vi "LH-01-17.vi"(0 "FPGA VI Reference In":refnum<k20>, 1 "OutputRange":cluster{"output high":dbl, "output low":dbl}[](array[cluster]), 2 "LHSetpoints":dbl[](array[numeric]), 3 "AIsLH":i32[](array[numeric]), 4 "error in":errorcluster, 6 "PIDs für \"träge\" Heizungen":T1(array[cluster])) -> (7 "error out":errorcluster)   [LabVIEW 2010]
uses:
  <vilib>/rvi/interface/nirviReadWriteControl/nirviReadWriteControl.xnode
  C:/Users/HAGAR-IV/Desktop/Zeugs/markus/version feb 2012/FPGA Bitfiles/pertrasgcfpga2_FPGATarget_FPGA-Programm-01_A75D3647.lvbitx
  C:/Users/HAGAR-IV/Desktop/Zeugs/Johnny/pertrasgc fpga/FPGA-Programm-01-17.vi
  <vilib>/rvi/interface/common/niFpgaNodeNameForErrorReporting.ctl
  <vilib>/rvi/errors/niLvFpgaWhatHappensToTopLevelVI.ctl
  GVHeizenLH.vi
  GVAIs.vi
  <vilib>/addons/control/pid/pid.llb/PID (DBL Array).vi
  <vilib>/Utility/error.llb/Error Cluster From Error Code.vi
  <vilib>/rvi/errors/niLvFpgaAdjustHostInterfaceError.vi
  <vilib>/addons/control/pid/NI_PID_pid.lvlib
  NiFpgaLv.dll
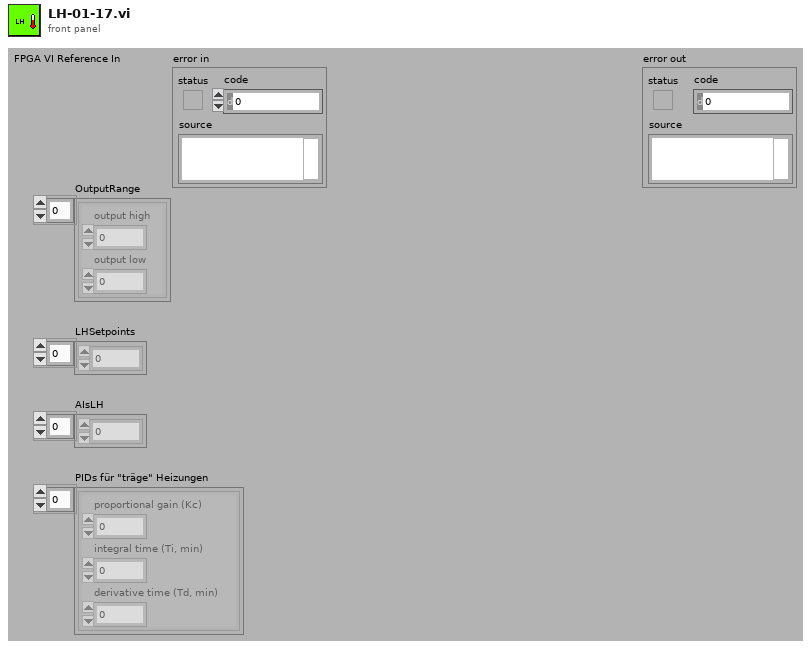
[diagram p1: front panel]
types:
  T1 = cluster{"proportional gain (Kc)":dbl, "integral time (Ti, min)":dbl, "derivative time (Td, min)":dbl}[]
  T2 = cluster{"Heizen?LH[0]":bool, "Heizen?LH[1]":bool, "Heizen?LH[2]":bool, "Heizen?LH[3]":bool, "Heizen?LH[4]":bool, "Heizen?LH[5]":bool, "Heizen?LH[6]":bool, "Heizen?LH[7]":bool, "Heizen?LH[8]":bool, "Heizen?LH[9]":bool, "Heizen?LH[10]":bool, "Heizen?LH[11]":bool}
  T3 = cluster{"[0]":u32, "[1]":u32, "[2]":u32, "[3]":u32, "[4]":u32, "[5]":u32, "[6]":u32, "[7]":u32, "[8]":u32, "[9]":u32, "[10]":u32, "[11]":u32}
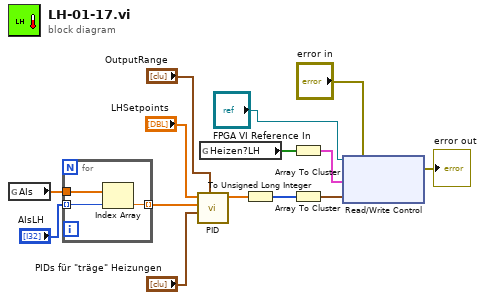
[diagram p0: block diagram]
diagram:
  n1 = global read "GVAIs.vi" "AIs"() -> (w12:dbl[])
  n2 = for {
    tunnel: w12 -> [w17]
    tunnel: "AIsLH" -> [w16] mode=indexing
    tunnel: [w15] -> w1 mode=indexing
    n3 = Index Array(array=w17, index=w16) -> (element=w15:dbl)
  }
  n4 = call-poly <vilib>:"PID.vi"("output range"="OutputRange", "PID gains"="PIDs für \"träge\" Heizungen", "process variable"=w1, "setpoint"="LHSetpoints") -> ("output"=w7:dbl[])  [unwired: 6 in, 1 out]
  n5 = global read "GVHeizenLH.vi" "Heizen?LH"() -> (w11:bool[])
  n6 = To Unsigned Long Integer(number=w7) -> (unsigned 32bit integer=w9:u32[])
  n7 = Array To Cluster(array=w11) -> (cluster=w8:T2)
  n8 = Array To Cluster(array=w9) -> (cluster=w10:T3)
  n9 = xnode "Read/Write Control"("FPGA VI Reference In"="FPGA VI Reference In", "error in"="error in", "LHHeizen?"=w8, "LHPulse(us)"=w10) -> ("error out"=→"error out":errorcluster)  [unwired: 1 out]
